vi "From 1D Int Tree Data.vi"(11 "Tree Data":refnum<class "Tree Data.lvclass">) -> (2 "1D Int":i64[](array[numeric]))   [LabVIEW 2017, in "Tree API.lvlib" / "1D Int.lvclass"]
doc: "Extract an 1D Int value from Tree Data type."
uses:
  1D Int.lvclass
  Tree Data/Tree Data.lvclass
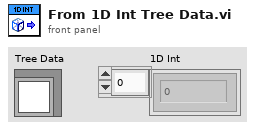
[diagram p1: front panel]
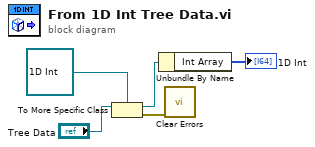
[diagram p0: block diagram]
diagram:
  n1 = To More Specific Class(target class=refnum<class "1D Int.lvclass"> refnum ("Int Array.lvclass"), reference="Tree Data") -> (specific class reference=w3:refnum<class "1D Int.lvclass">, error out=w4:errorcluster)  [unwired: 1 in]
  n2 = Unbundle By Name(w3) -> ("Int Array"=→"1D Int":i64[])
  n3 = call <vilib>:"Clear Errors.vi"("error in (no error)"=w4) -> ()  [unwired: 5 in, 2 out]
